vi "Format Type Name.vi"(10 "Pre-Name":string, 11 "Data Type":variant) -> (0 "error out":errorcluster, 2 "Name":string)   [LabVIEW 2015, in "Mediator.lvlib" / "Topic.lvclass"]
uses:
  Topic.lvclass
  <vilib>/Utility/Data Type/NI_Data Type.lvlib
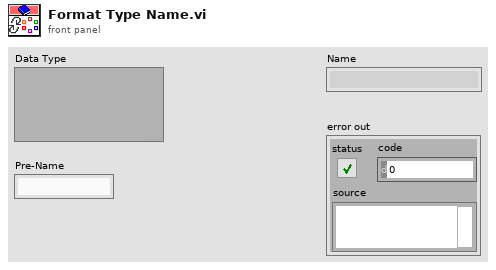
[diagram p1: front panel]
types:
  T1 = typedef "NI_Data Type.lvlib/Data Type.ctl" = enum8{"Invalid Type", "Void", "I8", "I16", "I32", "I64", "U8", "U16", "U32", "U64", "Single Float", "Double Float", "Extended Float", "Single Complex", "Double Complex", "Extended Complex", "Enum U8", "Enum U16", "Enum U32", "Enum U64", "Single Float With Unit", "Double Float With Unit", "Extended Float With Unit", "Single Complex with Unit", "Double Complex with Unit", "Extended Complex with Unit", "Boolean", "String", "Path", "Picture", "Tag", "Array", "Cluster", "Variant", "LV Variant", "Waveform", "Timestamp", "Digital Waveform", "Digital Data", "ExpressData", "Refnum", "External Data", "VI", "Poly VI", "LabVIEW Class Instance", "Fixed Point"}
  T2 = typedef "NI_Data Type.lvlib/Type Definition Info.ctl" = cluster{"Name":string, "Timestamp":u32}
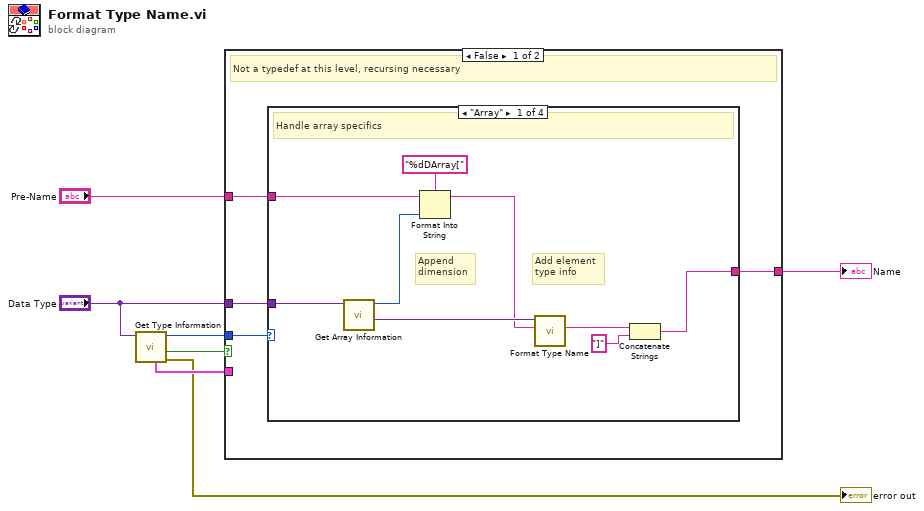
[diagram p0: block diagram]
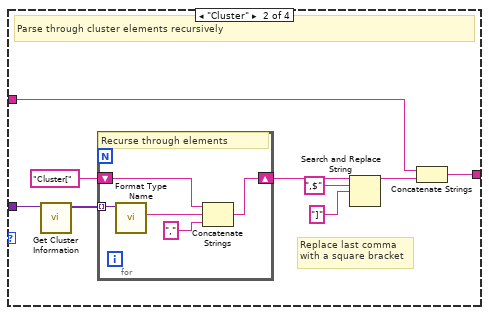
[diagram p2: hidden frame]
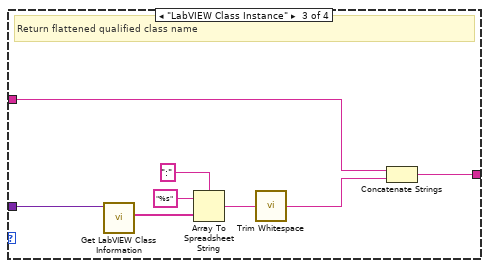
[diagram p3: hidden frame]
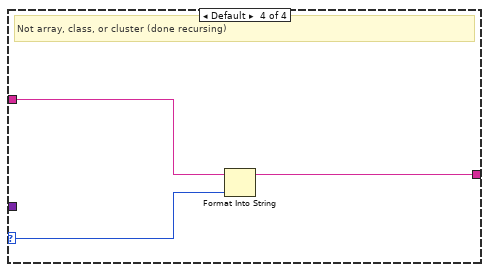
[diagram p4: hidden frame]
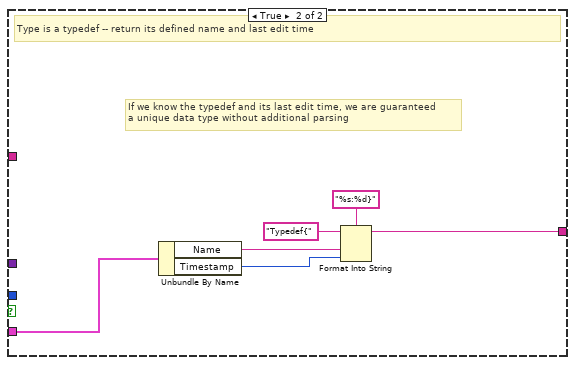
[diagram p5: hidden frame]
diagram:
  n1 = call <vilib>:"Get Type Information.vi"("Variant"="Data Type") -> ("error out"=→"error out":errorcluster, "Type Definition"=w4:bool, "Type"=w3:T1, "Type Definition Info"=w5:T2)  [unwired: 6 in, 1 out]
  n2 = case shown="False" w4 {
    tunnel: [w11 w47] -> w7
    tunnel: "Data Type" -> [w10 _]
    tunnel: "Pre-Name" -> [w9 _]
    tunnel: w3 -> [w8 _]
    tunnel: w5 -> [_ w51]
    frame False {
      # "Not a typedef at this level, recursing necessary"
      n3 = case shown="\"Array\"" w8 {
        selector: w8 -> [_ _ _ w45]
        tunnel: [w14 w26 w36 w43] -> w11
        tunnel: w10 -> [w20 w29 w42 _]
        tunnel: w9 -> [w19 w27 w35 w44]
        frame "Array" {
          # "Append\ndimension"
          # "Add element\ntype info"
          # "Handle array specifics"
          n4 = call <vilib>:"Get Array Information.vi"("Variant"=w20) -> ("Array Element Data Type"=w18:variant, "Number of Dimensions"=w16:i32)  [unwired: 7 in, 2 out]
          n5 = Format Into String(format string="%dDArray[", initial string=w19, w16) -> (resulting string=w12:string)  [unwired: 1 in, 1 out]
          n6 = call "Format Type Name.vi"("Pre-Name"=w12, "Data Type"=w18) -> ("Name"=w17:string)  [unwired: 8 in, 1 out]
          n7 = Concatenate Strings(w17, "]" ("string")) -> (w14:string)
        }
        frame "Cluster" {
          # "Replace last comma\nwith a square bracket"
          # "Parse through cluster elements recursively"
          n8 = call <vilib>:"Get Cluster Information.vi"("Variant"=w29) -> ("Cluster Elements"=w28:variant[])  [unwired: 9 in, 1 out]
          n9 = for {
            tunnel: w28 -> [w34] mode=indexing
            shift-right: [w32] -> w24
            shift-left: "Cluster[" ("string") -> [w30]
            # "Recurse through elements"
            n10 = call "Format Type Name.vi"("Data Type"=w34) -> ("Name"=w33:string)  [unwired: 9 in, 1 out]
            n11 = Concatenate Strings(w30, w33, "," ("string")) -> (w32:string)
          }
          n12 = Search and Replace String(input string=w24, search string=",$", replace string="]" ("string")) -> (result string=w21:string)  [unwired: 5 in, 3 out]
          n13 = Concatenate Strings(w27, w21) -> (w26:string)
        }
        frame "LabVIEW Class Instance" {
          # "Return flattened qualified class name"
          n14 = call <vilib>:"Get LabVIEW Class Information.vi"("Variant"=w42) -> ("Qualified LabVIEW Class Name"=w41:string[])  [unwired: 8 in, 2 out]
          n15 = Array To Spreadsheet String(delimiter (Tab)=":", array=w41, 3:"%s" ("format string")) -> (spreadsheet string=w38:string)
          n16 = call <vilib>:"Trim Whitespace.vi"("string"=w38) -> ("trimmed string"=w37:string)  [unwired: 1 in]
          n17 = Concatenate Strings(w35, w37) -> (w36:string)
        }
        frame Default {
          # "Not array, class, or cluster (done recursing)"
          n18 = Format Into String(initial string=w44, w45) -> (resulting string=w43:string)  [unwired: 2 in, 1 out]
        }
      }
    }
    frame True {
      # "If we know the typedef and its last edit time, we are guaranteed\na unique data type without additional parsing"
      # "Type is a typedef -- return its defined name and last edit time"
      n19 = Unbundle By Name(w51) -> ("Name"=w50:string, "Timestamp"=w46:u32)
      n20 = Format Into String(format string="%s:%d}", initial string="Typedef{", w50, w46) -> (resulting string=w47:string)  [unwired: 1 in, 1 out]
    }
  }
  "Name" <- w7
